vi "TDT-Init DAQ.vi"(0 "AO Fs (Hz)":dbl, 1 "Circuit":string, 2 "AI only":bool, 5 "AI Fs (Hz)":dbl, 7 "T (ms)":dbl, 9 "Num AO Buffers":i32=2, 11 "error in (no error)":errorcluster, 12 "AO Channels":i32[](array[numeric]), 13 "AI Channels":i32[](array[numeric])=[1, 2]) -> (4 "AO Fs (coerced)":dbl, 6 "AI Fs (coerced)":dbl, 8 "AO npts":i32, 10 "AI npts":i32, 15 "error out":errorcluster)   [LabVIEW 2020]
uses:
  TDT-Signal Bank Action.ctl
  TDT-Globals.vi
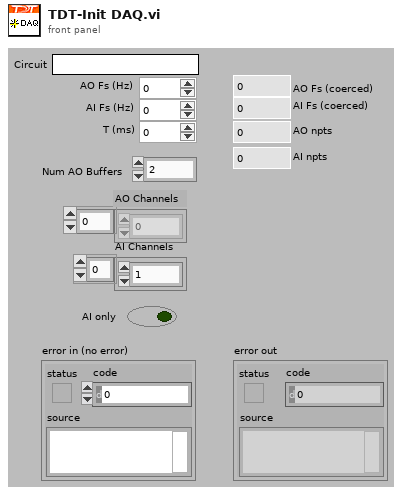
[diagram p1: front panel]
types:
  T1 = typedef "TDT-Signal Bank Action.ctl" = enum16{"Init", "Write", "Read", "Rewrite", "Reset", "Recycle", "Ramp up", "Ramp down", "Zero"}
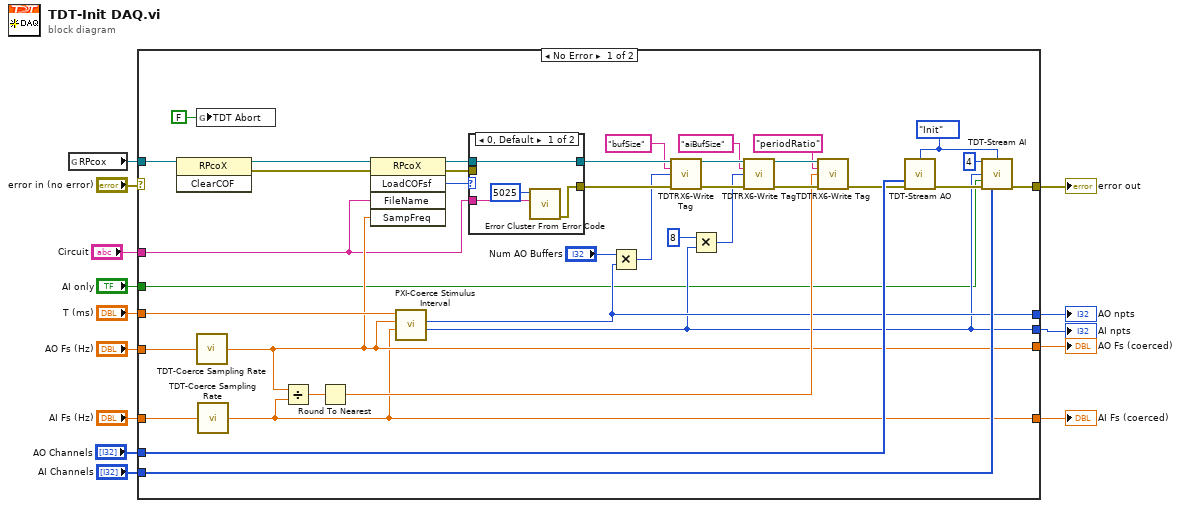
[diagram p0: block diagram]
diagram:
  n1 = global read "TDT-Globals.vi" "RPcox"() -> (w12:refnum<k7>)
  n2 = case shown="No Error" "error in (no error)" {
    selector: "error in (no error)" -> [_ w59]
    tunnel: [w35 w59] -> w13
    tunnel: w12 -> [w27 _]
    tunnel: "AO Fs (Hz)" -> [w37 _]
    tunnel: "AI Fs (Hz)" -> [w36 _]
    tunnel: "T (ms)" -> [w22 _]
    tunnel: [w21 _] -> w8
    tunnel: [w20 _] -> w7
    tunnel: [w19 _] -> w6
    tunnel: [w18 _] -> w5
    tunnel: "AI Channels" -> [w28 _]
    tunnel: "Circuit" -> [w15 _]
    tunnel: "AO Channels" -> [w24 _]
    tunnel: "AI only" -> [w16 _]
    frame No Error {
      w34 = TDT-Signal_Bank_Action."Init" ("Action")
      n3 = invoke class="RPcoX" method="ClearCOF"(reference=w27) -> (reference out=w26:refnum<k7>, error out=w25:errorcluster)  [unwired: 2 in, 1 out]
      n4 = global write "TDT-Globals.vi" "TDT Abort"(FALSE ("TDT Abort")) -> ()
      n5 = call "TDT-Coerce Sampling Rate.vi"("Fs (Hz)"=w37) -> ("Coerced"=w21:dbl)
      n6 = call "TDT-Coerce Sampling Rate.vi"("Fs (Hz)"=w36) -> ("Coerced"=w20:dbl)
      n7 = Divide(x=w21, y=w20) -> (x/y=w38:dbl)
      n8 = Round To Nearest(number=w38) -> (nearest integer value=w29:dbl)
      n9 = invoke class="RPcoX" method="LoadCOFsf"(reference=w26, error in=w25, "FileName"=w15, "SampFreq"=w21) -> (reference out=w51:refnum<k7>, error out=w50:errorcluster, "LoadCOFsf"=w52:i32)  [unwired: 1 in, 2 out]
      n10 = call "PXI-Coerce Stimulus Interval.vi"("AI sampling rate (Hz)"=w20, "AO sampling rate (Hz)"=w21, "Stimulus interval (ms)"=w22) -> ("AI npts"=w18:i32, "AO npts"=w19:i32)  [unwired: 5 in, 2 out]
      n11 = case shown="0, Default" w52 {
        tunnel: w15 -> [w55 _]
        tunnel: w51 -> [w56 w58]
        tunnel: w50 -> [_ w57]
        tunnel: [w56 w58] -> w49
        tunnel: [w53 w57] -> w48
        frame 0, Default {
          n12 = call <vilib>:"Error Cluster From Error Code.vi"("error message (\"\")"=w55, "error code (0)"=5025) -> ("error out"=w53:errorcluster)  [unwired: 7 in]
        }
        frame 1 {
        }
      }
      n13 = Multiply(x="Num AO Buffers", y=w19) -> (x*y=w31:i32)
      n14 = call "TDTRX6-Write Tag.vi"("RPcox"=w49, "Name"="bufSize", "Value"=w31, "error in"=w48) -> ("RPcox Out"=w45:refnum<k7>, "error out"=w46:errorcluster)  [unwired: 10 in]
      n15 = Multiply(x=8, y=w18) -> (x*y=w33:i32)
      n16 = call "TDTRX6-Write Tag.vi"("RPcox"=w45, "Name"="aiBufSize", "Value"=w33, "error in"=w46) -> ("RPcox Out"=w42:refnum<k7>, "error out"=w43:errorcluster)  [unwired: 10 in]
      n17 = call "TDTRX6-Write Tag.vi"("RPcox"=w42, "Name"="periodRatio", "Value"=w29, "error in"=w43) -> ("error out"=w23:errorcluster)  [unwired: 10 in, 1 out]
      n18 = call "TDT-Stream AO.vi"("Action"=w34, "Chans"=w24, "error in (no error)"=w23) -> ("error out"=w40:errorcluster)  [unwired: 12 in]
      n19 = call "TDT-Stream AI.vi"("#Inputs"=4, "Action"=w34, "Pts Per Read"=w18, "AI only"=w16, "error in (no error)"=w40, "AI Channels"=w28) -> ("error out"=w35:errorcluster)  [unwired: 8 in, 1 out]
    }
    frame Error {
    }
  }
  "error out" <- w13
  "AO Fs (coerced)" <- w8
  "AI Fs (coerced)" <- w7
  "AO npts" <- w6
  "AI npts" <- w5
